vi "CRYMain Close.vi"   [LabVIEW 2013]
panel:
  # "Main Close."
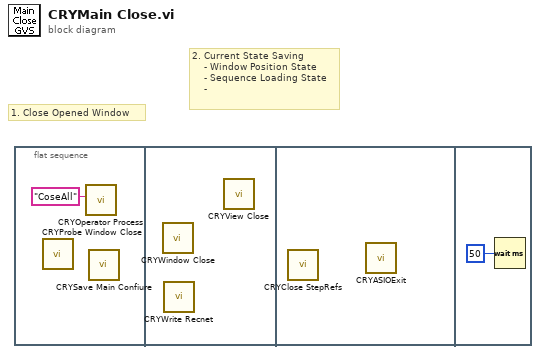
[diagram p0: block diagram]
diagram:
  # "2. Current State Saving\n    - Window Position State\n    - Sequence Loading State\n    -"
  # "1. Close Opened Window"
  n1 = flat-sequence {
    frame #0 {
      n2 = call "CRYProbe Window Close.vi"() -> ()  [unwired: 1 out]
      n3 = call "CRYOperator Process.vi"("sAction"="CoseAll") -> ()  [unwired: 10 in, 1 out]
      n4 = call "CRYSave Main Confiure.vi"() -> ()  [unwired: 1 out]
    }
    frame #1 {
      n5 = call "CRYWindow Close.vi"() -> ()  [unwired: 1 out]
      n6 = call "CRYWrite Recnet.vi"() -> ()  [unwired: 3 out]
      n7 = call "CRYView Close.vi"() -> ()  [unwired: 12 in]
    }
    frame #2 {
      n8 = call "CRYClose StepRefs.vi"() -> ()  [unwired: 12 in]
      n9 = call "CRYASIOExit.vi"() -> ()  [unwired: 10 in, 2 out]
    }
    frame #3 {
      n10 = Wait (ms)(milliseconds to wait=u32 50) -> ()  [unwired: 1 out]
    }
  }
